vi "StrToCode.vi"(11 "Name in":string="Name in") -> (3 "Name out":string)   [LabVIEW 2019]
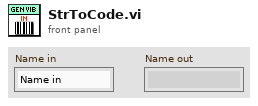
[diagram p1: front panel]
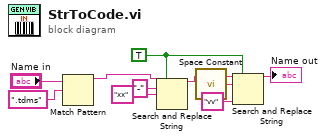
[diagram p0: block diagram]
diagram:
  w2 = TRUE ("replace all? (F)")
  n1 = Match Pattern(string="Name in", regular expression=".tdms") -> (before substring=w3:string)  [unwired: 1 in, 3 out]
  n2 = Search and Replace String(replace all?=w2, input string=w3, search string="-", replace string="xx" ("replace string (\"\")")) -> (result string=w7:string)  [unwired: 4 in, 3 out]
  n3 = call <vilib>:"Space Constant.vi"() -> ("String"=w6:string)
  n4 = Search and Replace String(replace all?=w2, input string=w7, search string=w6, replace string="vv" ("replace string (\"\")")) -> (result string=→"Name out":string)  [unwired: 4 in, 3 out]
